vi "Set Acc Time Param.vi"(8 "error in (no error)":errorcluster, 9 "DEC Time":i32, 10 "ACC Time":i32, 11 "FujiMotor in":refnum<class "FujiMotor.lvclass">) -> (0 "error out":errorcluster, 3 "FujiMotor out":refnum<class "FujiMotor.lvclass">)   [LabVIEW 2014, in "ALPHA5 RS485.lvlib" / "FujiMotor.lvclass"]
uses:
  FujiMotor.lvclass
  FujiMotor.lvclass/FujiMotor.ctl
  ALPHA5 RS485.lvlib
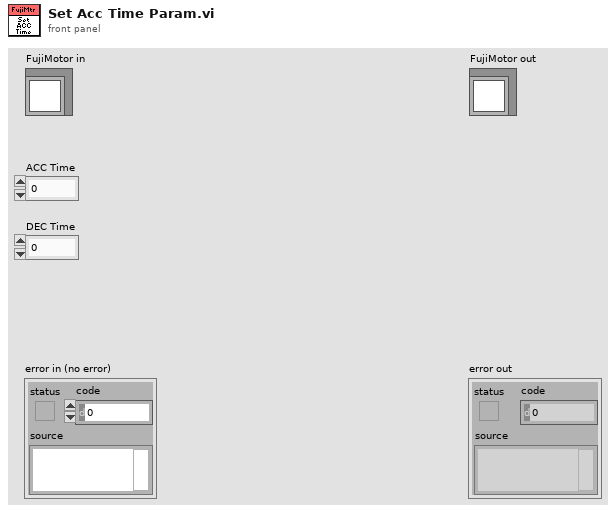
[diagram p1: front panel]
types:
  T1 = typedef "ALPHA5 RS485.lvlib/Port Selection Info.ctl" = cluster{"Port Name":refnum<visa-resource-name>, "Amplifier Num":u8, "Baud Rate":u32, "Char Formation":enum16{"0", "1", "2", "3", "4", "5"}}
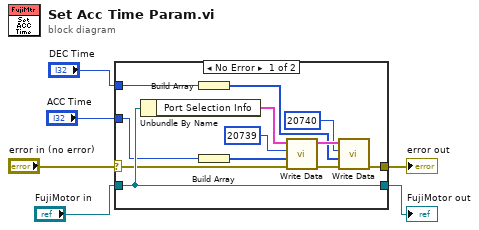
[diagram p0: block diagram]
diagram:
  n1 = case shown="No Error" "error in (no error)" {
    selector: "error in (no error)" -> [w8 w19]
    tunnel: [w7 w19] -> w5
    tunnel: [w18 w20] -> w3
    tunnel: "FujiMotor in" -> [w18 w20]
    tunnel: "ACC Time" -> [w15 _]
    tunnel: "DEC Time" -> [w10 _]
    frame No Error {
      n2 = Unbundle By Name(w18) -> ("Port Selection Info"=w17:T1)
      n3 = Build Array(w10) -> (w9:i32[])
      n4 = Build Array(w15) -> (w16:i32[])
      n5 = call "Write Data.vi"("error in (no error)"=w8, "Data"=w16, "Address"=u16 20739, "Port Selection Info In"=w17) -> ("error out"=w13:errorcluster, "Port Selection Info Out"=w12:T1)  [unwired: 6 in]
      n6 = call "Write Data.vi"("error in (no error)"=w13, "Data"=w9, "Address"=u16 20740, "Port Selection Info In"=w12) -> ("error out"=w7:errorcluster)  [unwired: 6 in, 1 out]
    }
    frame Error {
    }
  }
  "error out" <- w5
  "FujiMotor out" <- w3
